vi "App - analyze RUS V6.vi"() -> ()   [LabVIEW 2021] (continued)
"mod time(min)"=58231368.86666667, "file format"=enum."binary", "power(V)"=2.1, "Magn Field(T) "=0.0}, {"temperature"=14.481, "temperature str"="14.48100", "file path"=path "D:/Data/Ultrasound/LSCO/LSCO22__130814c/5_Cooling_2nd_try/September_2014/091814/14.48100K_500_2500_2.10000V_0.00000T_Sep18-2014__06-50-12_001_091814.bin", "last mod"=timestamp(3493882212 s since 1904-01-01), "file name str"="D:\\Data\\Ultrasound\\LSCO\\LSCO22__130814c\\5_Cooling_2nd_try\\September_2014\\091814\\14.48100K_500_2500_2.10000V_0.00000T_Sep18-2014__06-50-12_001_091814.bin", "mod time(min)"=58231370.2, "file format"=enum."binary", "power(V)"=2.1, "Magn Field(T) "=0.0}, {"temperature"=14.483, "temperature str"="14.48300", "file path"=path "D:/Data/Ultrasound/LSCO/LSCO22__130814c/5_Cooling_2nd_try/September_2014/091814/14.48300K_500_2500_2.10000V_0.00000T_Sep18-2014__06-51-31_001_091814.bin", "last mod"=timestamp(3493882291 s since 1904-01-01), "file name str"="D:\\Data\\Ultrasound\\LSCO\\LSCO22__130814c\\5_Cooling_2nd_try\\September_2014\\091814\\14.48300K_500_2500_2.10000V_0.00000T_Sep18-2014__06-51-31_001_091814.bin", "mod time(min)"=58231371.516666666, "file format"=enum."binary", "power(V)"=2.1, "Magn Field(T) "=0.0}, {"temperature"=14.483, "temperature str"="14.48300", "file path"=path "D:/Data/Ultrasound/LSCO/LSCO22__130814c/5_Cooling_2nd_try/September_2014/091814/14.48300K_500_2500_2.10000V_0.00000T_Sep18-2014__06-52-50_001_091814.bin", "last mod"=timestamp(3493882370 s since 1904-01-01), "file name str"="D:\\Data\\Ultrasound\\LSCO\\LSCO22__130814c\\5_Cooling_2nd_try\\September_2014\\091814\\14.48300K_500_2500_2.10000V_0.00000T_Sep18-2014__06-52-50_001_091814.bin", "mod time(min)"=58231372.833333336, "file format"=enum."binary", "power(V)"=2.1, "Magn Field(T) "=0.0}, {"temperature"=14.484, "temperature str"="14.48400", "file path"=path "D:/Data/Ultrasound/LSCO/LSCO22__130814c/5_Cooling_2nd_try/September_2014/091814/14.48400K_500_2500_2.10000V_0.00000T_Sep18-2014__06-54-10_001_091814.bin", "last mod"=timestamp(3493882450 s since 1904-01-01), "file name str"="D:\\Data\\Ultrasound\\LSCO\\LSCO22__130814c\\5_Cooling_2nd_try\\September_2014\\091814\\14.48400K_500_2500_2.10000V_0.00000T_Sep18-2014__06-54-10_001_091814.bin", "mod time(min)"=58231374.166666664, "file format"=enum."binary", "power(V)"=2.1, "Magn Field(T) "=0.0}, {"temperature"=14.488, "temperature str"="14.48800", "file path"=path "D:/Data/Ultrasound/LSCO/LSCO22__130814c/5_Cooling_2nd_try/September_2014/091814/14.48800K_500_2500_2.10000V_0.00000T_Sep18-2014__06-55-29_001_091814.bin", "last mod"=timestamp(3493882529 s since 1904-01-01), "file name str"="D:\\Data\\Ultrasound\\LSCO\\LSCO22__130814c\\5_Cooling_2nd_try\\September_2014\\091814\\14.48800K_500_2500_2.10000V_0.00000T_Sep18-2014__06-55-29_001_091814.bin", "mod time(min)"=58231375.483333334, "file format"=enum."binary", "power(V)"=2.1, "Magn Field(T) "=0.0}, {"temperature"=14.49, "temperature str"="14.49000", "file path"=path "D:/Data/Ultrasound/LSCO/LSCO22__130814c/5_Cooling_2nd_try/September_2014/091814/14.49000K_500_2500_2.10000V_0.00000T_Sep18-2014__06-56-49_001_091814.bin", "last mod"=timestamp(3493882609 s since 1904-01-01), "file name str"="D:\\Data\\Ultrasound\\LSCO\\LSCO22__130814c\\5_Cooling_2nd_try\\September_2014\\091814\\14.49000K_500_2500_2.10000V_0.00000T_Sep18-2014__06-56-49_001_091814.bin", "mod time(min)"=58231376.81666667, "file format"=enum."binary", "power(V)"=2.1, "Magn Field(T) "=0.0}, {"temperature"=14.491, "temperature str"="14.49100", "file path"=path "D:/Data/Ultrasound/LSCO/LSCO22__130814c/5_Cooling_2nd_try/September_2014/091814/14.49100K_500_2500_2.10000V_0.00000T_Sep18-2014__06-58-08_001_091814.bin", "last mod"=timestamp(3493882688 s since 1904-01-01), "file name str"="D:\\Data\\Ultrasound\\LSCO\\LSCO22__130814c\\5_Cooling_2nd_try\\September_2014\\091814\\14.49100K_500_2500_2.10000V_0.00000T_Sep18-2014__06-58-08_001_091814.bin", "mod time(min)"=58231378.13333333, "file format"=enum."binary", "power(V)"=2.1, "Magn Field(T) "=0.0}, {"temperature"=14.493, "temperature str"="14.49300", "file path"=path "D:/Data/Ultrasound/LSCO/LSCO22__130814c/5_Cooling_2nd_try/September_2014/091814/14.49300K_500_2500_2.10000V_0.00000T_Sep18-2014__06-59-27_001_091814.bin", "last mod"=timestamp(3493882767 s since 1904-01-01), "file name str"="D:\\Data\\Ultrasound\\LSCO\\LSCO22__130814c\\5_Cooling_2nd_try\\September_2014\\091814\\14.49300K_500_2500_2.10000V_0.00000T_Sep18-2014__06-59-27_001_091814.bin", "mod time(min)"=58231379.45, "file format"=enum."binary", "power(V)"=2.1, "Magn Field(T) "=0.0}, {"temperature"=14.491, "temperature str"="14.49100", "file path"=path "D:/Data/Ultrasound/LSCO/LSCO22__130814c/5_Cooling_2nd_try/September_2014/091814/14.49100K_500_2500_2.10000V_0.00000T_Sep18-2014__07-00-47_001_091814.bin", "last mod"=timestamp(3493882847 s since 1904-01-01), "file name str"="D:\\Data\\Ultrasound\\LSCO\\LSCO22__130814c\\5_Cooling_2nd_try\\September_2014\\091814\\14.49100K_500_2500_2.10000V_0.00000T_Sep18-2014__07-00-47_001_091814.bin", "mod time(min)"=58231380.78333333, "file format"=enum."binary", "power(V)"=2.1, "Magn Field(T) "=0.0}, {"temperature"=14.489, "temperature str"="14.48900", "file path"=path "D:/Data/Ultrasound/LSCO/LSCO22__130814c/5_Cooling_2nd_try/September_2014/091814/14.48900K_500_2500_2.10000V_0.00000T_Sep18-2014__07-02-06_001_091814.bin", "last mod"=timestamp(3493882926 s since 1904-01-01), "file name str"="D:\\Data\\Ultrasound\\LSCO\\LSCO22__130814c\\5_Cooling_2nd_try\\September_2014\\091814\\14.48900K_500_2500_2.10000V_0.00000T_Sep18-2014__07-02-06_001_091814.bin", "mod time(min)"=58231382.1, "file format"=enum."binary", "power(V)"=2.1, "Magn Field(T) "=0.0}, {"temperature"=14.491, "temperature str"="14.49100", "file path"=path "D:/Data/Ultrasound/LSCO/LSCO22__130814c/5_Cooling_2nd_try/September_2014/091814/14.49100K_500_2500_2.10000V_0.00000T_Sep18-2014__07-03-26_001_091814.bin", "last mod"=timestamp(3493883006 s since 1904-01-01), "file name str"="D:\\Data\\Ultrasound\\LSCO\\LSCO22__130814c\\5_Cooling_2nd_try\\September_2014\\091814\\14.49100K_500_2500_2.10000V_0.00000T_Sep18-2014__07-03-26_001_091814.bin", "mod time(min)"=58231383.43333333, "file format"=enum."binary", "power(V)"=2.1, "Magn Field(T) "=0.0}, {"temperature"=14.492, "temperature str"="14.49200", "file path"=path "D:/Data/Ultrasound/LSCO/LSCO22__130814c/5_Cooling_2nd_try/September_2014/091814/14.49200K_500_2500_2.10000V_0.00000T_Sep18-2014__07-04-45_001_091814.bin", "last mod"=timestamp(3493883085 s since 1904-01-01), "file name str"="D:\\Data\\Ultrasound\\LSCO\\LSCO22__130814c\\5_Cooling_2nd_try\\September_2014\\091814\\14.49200K_500_2500_2.10000V_0.00000T_Sep18-2014__07-04-45_001_091814.bin", "mod time(min)"=58231384.75, "file format"=enum."binary", "power(V)"=2.1, "Magn Field(T) "=0.0}, {"temperature"=14.492, "temperature str"="14.49200", "file path"=path "D:/Data/Ultrasound/LSCO/LSCO22__130814c/5_Cooling_2nd_try/September_2014/091814/14.49200K_500_2500_2.10000V_0.00000T_Sep18-2014__07-06-04_001_091814.bin", "last mod"=timestamp(3493883164 s since 1904-01-01), "file name str"="D:\\Data\\Ultrasound\\LSCO\\LSCO22__130814c\\5_Cooling_2nd_try\\September_2014\\091814\\14.49200K_500_2500_2.10000V_0.00000T_Sep18-2014__07-06-04_001_091814.bin", "mod time(min)"=58231386.06666667, "file format"=enum."binary", "power(V)"=2.1, "Magn Field(T) "=0.0}, {"temperature"=14.496, "temperature str"="14.49600", "file path"=path "D:/Data/Ultrasound/LSCO/LSCO22__130814c/5_Cooling_2nd_try/September_2014/091814/14.49600K_500_2500_2.10000V_0.00000T_Sep18-2014__07-07-24_001_091814.bin", "last mod"=timestamp(3493883244 s since 1904-01-01), "file name str"="D:\\Data\\Ultrasound\\LSCO\\LSCO22__130814c\\5_Cooling_2nd_try\\September_2014\\091814\\14.49600K_500_2500_2.10000V_0.00000T_Sep18-2014__07-07-24_001_091814.bin", "mod time(min)"=58231387.4, "file format"=enum."binary", "power(V)"=2.1, "Magn Field(T) "=0.0}, {"temperature"=14.498, "temperature str"="14.49800", "file path"=path "D:/Data/Ultrasound/LSCO/LSCO22__130814c/5_Cooling_2nd_try/September_2014/091814/14.49800K_500_2500_2.10000V_0.00000T_Sep18-2014__07-08-43_001_091814.bin", "last mod"=timestamp(3493883323 s since 1904-01-01), "file name str"="D:\\Data\\Ultrasound\\LSCO\\LSCO22__130814c\\5_Cooling_2nd_try\\September_2014\\091814\\14.49800K_500_2500_2.10000V_0.00000T_Sep18-2014__07-08-43_001_091814.bin", "mod time(min)"=58231388.71666667, "file format"=enum."binary", "power(V)"=2.1, "Magn Field(T) "=0.0}, {"temperature"=14.495, "temperature str"="14.49500", "file path"=path "D:/Data/Ultrasound/LSCO/LSCO22__130814c/5_Cooling_2nd_try/September_2014/091814/14.49500K_500_2500_2.10000V_0.00000T_Sep18-2014__07-10-02_001_091814.bin", "last mod"=timestamp(3493883402 s since 1904-01-01), "file name str"="D:\\Data\\Ultrasound\\LSCO\\LSCO22__130814c\\5_Cooling_2nd_try\\September_2014\\091814\\14.49500K_500_2500_2.10000V_0.00000T_Sep18-2014__07-10-02_001_091814.bin", "mod time(min)"=58231390.03333333, "file format"=enum."binary", "power(V)"=2.1, "Magn Field(T) "=0.0}, {"temperature"=14.498, "temperature str"="14.49800", "file path"=path "D:/Data/Ultrasound/LSCO/LSCO22__130814c/5_Cooling_2nd_try/September_2014/091814/14.49800K_500_2500_2.10000V_0.00000T_Sep18-2014__07-11-22_001_091814.bin", "last mod"=timestamp(3493883482 s since 1904-01-01), "file name str"="D:\\Data\\Ultrasound\\LSCO\\LSCO22__130814c\\5_Cooling_2nd_try\\September_2014\\091814\\14.49800K_500_2500_2.10000V_0.00000T_Sep18-2014__07-11-22_001_091814.bin", "mod time(min)"=58231391.36666667, "file format"=enum."binary", "power(V)"=2.1, "Magn Field(T) "=0.0}, {"temperature"=14.496, "temperature str"="14.49600", "file path"=path "D:/Data/Ultrasound/LSCO/LSCO22__130814c/5_Cooling_2nd_try/September_2014/091814/14.49600K_500_2500_2.10000V_0.00000T_Sep18-2014__07-12-41_001_091814.bin", "last mod"=timestamp(3493883561 s since 1904-01-01), "file name str"="D:\\Data\\Ultrasound\\LSCO\\LSCO22__130814c\\5_Cooling_2nd_try\\September_2014\\091814\\14.49600K_500_2500_2.10000V_0.00000T_Sep18-2014__07-12-41_001_091814.bin", "mod time(min)"=58231392.68333333, "file format"=enum."binary", "power(V)"=2.1, "Magn Field(T) "=0.0}, {"temperature"=14.503, "temperature str"="14.50300", "file path"=path "D:/Data/Ultrasound/LSCO/LSCO22__130814c/5_Cooling_2nd_try/September_2014/091814/14.50300K_500_2500_2.10000V_0.00000T_Sep18-2014__07-14-01_001_091814.bin", "last mod"=timestamp(3493883641 s since 1904-01-01), "file name str"="D:\\Data\\Ultrasound\\LSCO\\LSCO22__130814c\\5_Cooling_2nd_try\\September_2014\\091814\\14.50300K_500_2500_2.10000V_0.00000T_Sep18-2014__07-14-01_001_091814.bin", "mod time(min)"=58231394.016666666, "file format"=enum."binary", "power(V)"=2.1, "Magn Field(T) "=0.0}, {"temperature"=14.504, "temperature str"="14.50400", "file path"=path "D:/Data/Ultrasound/LSCO/LSCO22__130814c/5_Cooling_2nd_try/September_2014/091814/14.50400K_500_2500_2.10000V_0.00000T_Sep18-2014__07-15-20_001_091814.bin", "last mod"=timestamp(3493883720 s since 1904-01-01), "file name str"="D:\\Data\\Ultrasound\\LSCO\\LSCO22__130814c\\5_Cooling_2nd_try\\September_2014\\091814\\14.50400K_500_2500_2.10000V_0.00000T_Sep18-2014__07-15-20_001_091814.bin", "mod time(min)"=58231395.333333336, "file format"=enum."binary", "power(V)"=2.1, "Magn Field(T) "=0.0}, {"temperature"=14.507, "temperature str"="14.50700", "file path"=path "D:/Data/Ultrasound/LSCO/LSCO22__130814c/5_Cooling_2nd_try/September_2014/091814/14.50700K_500_2500_2.10000V_0.00000T_Sep18-2014__07-16-39_001_091814.bin", "last mod"=timestamp(3493883799 s since 1904-01-01), "file name str"="D:\\Data\\Ultrasound\\LSCO\\LSCO22__130814c\\5_Cooling_2nd_try\\September_2014\\091814\\14.50700K_500_2500_2.10000V_0.00000T_Sep18-2014__07-16-39_001_091814.bin", "mod time(min)"=58231396.65, "file format"=enum."binary", "power(V)"=2.1, "Magn Field(T) "=0.0}, {"temperature"=14.507, "temperature str"="14.50700", "file path"=path "D:/Data/Ultrasound/LSCO/LSCO22__130814c/5_Cooling_2nd_try/September_2014/091814/14.50700K_500_2500_2.10000V_0.00000T_Sep18-2014__07-17-59_001_091814.bin", "last mod"=timestamp(3493883879 s since 1904-01-01), "file name str"="D:\\Data\\Ultrasound\\LSCO\\LSCO22__130814c\\5_Cooling_2nd_try\\September_2014\\091814\\14.50700K_500_2500_2.10000V_0.00000T_Sep18-2014__07-17-59_001_091814.bin", "mod time(min)"=58231397.983333334, "file format"=enum."binary", "power(V)"=2.1, "Magn Field(T) "=0.0}, {"temperature"=14.508, "temperature str"="14.50800", "file path"=path "D:/Data/Ultrasound/LSCO/LSCO22__130814c/5_Cooling_2nd_try/September_2014/091814/14.50800K_500_2500_2.10000V_0.00000T_Sep18-2014__07-19-18_001_091814.bin", "last mod"=timestamp(3493883958 s since 1904-01-01), "file name str"="D:\\Data\\Ultrasound\\LSCO\\LSCO22__130814c\\5_Cooling_2nd_try\\September_2014\\091814\\14.50800K_500_2500_2.10000V_0.00000T_Sep18-2014__07-19-18_001_091814.bin", "mod time(min)"=58231399.3, "file format"=enum."binary", "power(V)"=2.1, "Magn Field(T) "=0.0}, {"temperature"=14.507, "temperature str"="14.50700", "file path"=path "D:/Data/Ultrasound/LSCO/LSCO22__130814c/5_Cooling_2nd_try/September_2014/091814/14.50700K_500_2500_2.10000V_0.00000T_Sep18-2014__07-20-37_001_091814.bin", "last mod"=timestamp(3493884037 s since 1904-01-01), "file name str"="D:\\Data\\Ultrasound\\LSCO\\LSCO22__130814c\\5_Cooling_2nd_try\\September_2014\\091814\\14.50700K_500_2500_2.10000V_0.00000T_Sep18-2014__07-20-37_001_091814.bin", "mod time(min)"=58231400.61666667, "file format"=enum."binary", "power(V)"=2.1, "Magn Field(T) "=0.0}, {"temperature"=14.507, "temperature str"="14.50700", "file path"=path "D:/Data/Ultrasound/LSCO/LSCO22__130814c/5_Cooling_2nd_try/September_2014/091814/14.50700K_500_2500_2.10000V_0.00000T_Sep18-2014__07-21-57_001_091814.bin", "last mod"=timestamp(3493884117 s since 1904-01-01), "file name str"="D:\\Data\\Ultrasound\\LSCO\\LSCO22__130814c\\5_Cooling_2nd_try\\September_2014\\091814\\14.50700K_500_2500_2.10000V_0.00000T_Sep18-2014__07-21-57_001_091814.bin", "mod time(min)"=58231401.95, "file format"=enum."binary", "power(V)"=2.1, "Magn Field(T) "=0.0}, {"temperature"=14.508, "temperature str"="14.50800", "file path"=path "D:/Data/Ultrasound/LSCO/LSCO22__130814c/5_Cooling_2nd_try/September_2014/091814/14.50800K_500_2500_2.10000V_0.00000T_Sep18-2014__07-23-16_001_091814.bin", "last mod"=timestamp(3493884196 s since 1904-01-01), "file name str"="D:\\Data\\Ultrasound\\LSCO\\LSCO22__130814c\\5_Cooling_2nd_try\\September_2014\\091814\\14.50800K_500_2500_2.10000V_0.00000T_Sep18-2014__07-23-16_001_091814.bin", "mod time(min)"=58231403.266666666, "file format"=enum."binary", "power(V)"=2.1, "Magn Field(T) "=0.0}, {"temperature"=14.509, "temperature str"="14.50900", "file path"=path "D:/Data/Ultrasound/LSCO/LSCO22__130814c/5_Cooling_2nd_try/September_2014/091814/14.50900K_500_2500_2.10000V_0.00000T_Sep18-2014__07-24-36_001_091814.bin", "last mod"=timestamp(3493884276 s since 1904-01-01), "file name str"="D:\\Data\\Ultrasound\\LSCO\\LSCO22__130814c\\5_Cooling_2nd_try\\September_2014\\091814\\14.50900K_500_2500_2.10000V_0.00000T_Sep18-2014__07-24-36_001_091814.bin", "mod time(min)"=58231404.6, "file format"=enum."binary", "power(V)"=2.1, "Magn Field(T) "=0.0}, {"temperature"=14.511, "temperature str"="14.51100", "file path"=path "D:/Data/Ultrasound/LSCO/LSCO22__130814c/5_Cooling_2nd_try/September_2014/091814/14.51100K_500_2500_2.10000V_0.00000T_Sep18-2014__07-25-55_001_091814.bin", "last mod"=timestamp(3493884355 s since 1904-01-01), "file name str"="D:\\Data\\Ultrasound\\LSCO\\LSCO22__130814c\\5_Cooling_2nd_try\\September_2014\\091814\\14.51100K_500_2500_2.10000V_0.00000T_Sep18-2014__07-25-55_001_091814.bin", "mod time(min)"=58231405.916666664, "file format"=enum."binary", "power(V)"=2.1, "Magn Field(T) "=0.0}, {"temperature"=14.513, "temperature str"="14.51300", "file path"=path "D:/Data/Ultrasound/LSCO/LSCO22__130814c/5_Cooling_2nd_try/September_2014/091814/14.51300K_500_2500_2.10000V_0.00000T_Sep18-2014__07-27-14_001_091814.bin", "last mod"=timestamp(3493884434 s since 1904-01-01), "file name str"="D:\\Data\\Ultrasound\\LSCO\\LSCO22__130814c\\5_Cooling_2nd_try\\September_2014\\091814\\14.51300K_500_2500_2.10000V_0.00000T_Sep18-2014__07-27-14_001_091814.bin", "mod time(min)"=58231407.233333334, "file format"=enum."binary", "power(V)"=2.1, "Magn Field(T) "=0.0}, {"temperature"=14.511, "temperature str"="14.51100", "file path"=path "D:/Data/Ultrasound/LSCO/LSCO22__130814c/5_Cooling_2nd_try/September_2014/091814/14.51100K_500_2500_2.10000V_0.00000T_Sep18-2014__07-28-34_001_091814.bin", "last mod"=timestamp(3493884514 s since 1904-01-01), "file name str"="D:\\Data\\Ultrasound\\LSCO\\LSCO22__130814c\\5_Cooling_2nd_try\\September_2014\\091814\\14.51100K_500_2500_2.10000V_0.00000T_Sep18-2014__07-28-34_001_091814.bin", "mod time(min)"=58231408.56666667, "file format"=enum."binary", "power(V)"=2.1, "Magn Field(T) "=0.0}, {"temperature"=14.512, "temperature str"="14.51200", "file path"=path "D:/Data/Ultrasound/LSCO/LSCO22__130814c/5_Cooling_2nd_try/September_2014/091814/14.51200K_500_2500_2.10000V_0.00000T_Sep18-2014__07-29-53_001_091814.bin", "last mod"=timestamp(3493884593 s since 1904-01-01), "file name str"="D:\\Data\\Ultrasound\\LSCO\\LSCO22__130814c\\5_Cooling_2nd_try\\September_2014\\091814\\14.51200K_500_2500_2.10000V_0.00000T_Sep18-2014__07-29-53_001_091814.bin", "mod time(min)"=58231409.88333333, "file format"=enum."binary", "power(V)"=2.1, "Magn Field(T) "=0.0}, {"temperature"=14.512, "temperature str"="14.51200", "file path"=path "D:/Data/Ultrasound/LSCO/LSCO22__130814c/5_Cooling_2nd_try/September_2014/091814/14.51200K_500_2500_2.10000V_0.00000T_Sep18-2014__07-31-13_001_091814.bin", "last mod"=timestamp(3493884673 s since 1904-01-01), "file name str"="D:\\Data\\Ultrasound\\LSCO\\LSCO22__130814c\\5_Cooling_2nd_try\\September_2014\\091814\\14.51200K_500_2500_2.10000V_0.00000T_Sep18-2014__07-31-13_001_091814.bin", "mod time(min)"=58231411.21666667, "file format"=enum."binary", "power(V)"=2.1, "Magn Field(T) "=0.0}, {"temperature"=14.51, "temperature str"="14.51000", "file path"=path "D:/Data/Ultrasound/LSCO/LSCO22__130814c/5_Cooling_2nd_try/September_2014/091814/14.51000K_500_2500_2.10000V_0.00000T_Sep18-2014__07-32-32_001_091814.bin", "last mod"=timestamp(3493884752 s since 1904-01-01), "file name str"="D:\\Data\\Ultrasound\\LSCO\\LSCO22__130814c\\5_Cooling_2nd_try\\September_2014\\091814\\14.51000K_500_2500_2.10000V_0.00000T_Sep18-2014__07-32-32_001_091814.bin", "mod time(min)"=58231412.53333333, "file format"=enum."binary", "power(V)"=2.1, "Magn Field(T) "=0.0}, {"temperature"=14.511, "temperature str"="14.51100", "file path"=path "D:/Data/Ultrasound/LSCO/LSCO22__130814c/5_Cooling_2nd_try/September_2014/091814/14.51100K_500_2500_2.10000V_0.00000T_Sep18-2014__07-33-51_001_091814.bin", "last mod"=timestamp(3493884831 s since 1904-01-01), "file name str"="D:\\Data\\Ultrasound\\LSCO\\LSCO22__130814c\\5_Cooling_2nd_try\\September_2014\\091814\\14.51100K_500_2500_2.10000V_0.00000T_Sep18-2014__07-33-51_001_091814.bin", "mod time(min)"=58231413.85, "file format"=enum."binary", "power(V)"=2.1, "Magn Field(T) "=0.0}, {"temperature"=14.511, "temperature str"="14.51100", "file path"=path "D:/Data/Ultrasound/LSCO/LSCO22__130814c/5_Cooling_2nd_try/September_2014/091814/14.51100K_500_2500_2.10000V_0.00000T_Sep18-2014__07-35-11_001_091814.bin", "last mod"=timestamp(3493884911 s since 1904-01-01), "file name str"="D:\\Data\\Ultrasound\\LSCO\\LSCO22__130814c\\5_Cooling_2nd_try\\September_2014\\091814\\14.51100K_500_2500_2.10000V_0.00000T_Sep18-2014__07-35-11_001_091814.bin", "mod time(min)"=58231415.18333333, "file format"=enum."binary", "power(V)"=2.1, "Magn Field(T) "=0.0}, {"temperature"=14.511, "temperature str"="14.51100", "file path"=path "D:/Data/Ultrasound/LSCO/LSCO22__130814c/5_Cooling_2nd_try/September_2014/091814/14.51100K_500_2500_2.10000V_0.00000T_Sep18-2014__07-36-30_001_091814.bin", "last mod"=timestamp(3493884990 s since 1904-01-01), "file name str"="D:\\Data\\Ultrasound\\LSCO\\LSCO22__130814c\\5_Cooling_2nd_try\\September_2014\\091814\\14.51100K_500_2500_2.10000V_0.00000T_Sep18-2014__07-36-30_001_091814.bin", "mod time(min)"=58231416.5, "file format"=enum."binary", "power(V)"=2.1, "Magn Field(T) "=0.0}, {"temperature"=14.512, "temperature str"="14.51200", "file path"=path "D:/Data/Ultrasound/LSCO/LSCO22__130814c/5_Cooling_2nd_try/September_2014/091814/14.51200K_500_2500_2.10000V_0.00000T_Sep18-2014__07-37-49_001_091814.bin", "last mod"=timestamp(3493885069 s since 1904-01-01), "file name str"="D:\\Data\\Ultrasound\\LSCO\\LSCO22__130814c\\5_Cooling_2nd_try\\September_2014\\091814\\14.51200K_500_2500_2.10000V_0.00000T_Sep18-2014__07-37-49_001_091814.bin", "mod time(min)"=58231417.81666667, "file format"=enum."binary", "power(V)"=2.1, "Magn Field(T) "=0.0}, {"temperature"=14.517, "temperature str"="14.51700", "file path"=path "D:/Data/Ultrasound/LSCO/LSCO22__130814c/5_Cooling_2nd_try/September_2014/091814/14.51700K_500_2500_2.10000V_0.00000T_Sep18-2014__07-39-09_001_091814.bin", "last mod"=timestamp(3493885149 s since 1904-01-01), "file name str"="D:\\Data\\Ultrasound\\LSCO\\LSCO22__130814c\\5_Cooling_2nd_try\\September_2014\\091814\\14.51700K_500_2500_2.10000V_0.00000T_Sep18-2014__07-39-09_001_091814.bin", "mod time(min)"=58231419.15, "file format"=enum."binary", "power(V)"=2.1, "Magn Field(T) "=0.0}, {"temperature"=14.515, "temperature str"="14.51500", "file path"=path "D:/Data/Ultrasound/LSCO/LSCO22__130814c/5_Cooling_2nd_try/September_2014/091814/14.51500K_500_2500_2.10000V_0.00000T_Sep18-2014__07-40-28_001_091814.bin", "last mod"=timestamp(3493885228 s since 1904-01-01), "file name str"="D:\\Data\\Ultrasound\\LSCO\\LSCO22__130814c\\5_Cooling_2nd_try\\September_2014\\091814\\14.51500K_500_2500_2.10000V_0.00000T_Sep18-2014__07-40-28_001_091814.bin", "mod time(min)"=58231420.46666667, "file format"=enum."binary", "power(V)"=2.1, "Magn Field(T) "=0.0}, {"temperature"=14.518, "temperature str"="14.51800", "file path"=path "D:/Data/Ultrasound/LSCO/LSCO22__130814c/5_Cooling_2nd_try/September_2014/091814/14.51800K_500_2500_2.10000V_0.00000T_Sep18-2014__07-41-48_001_091814.bin", "last mod"=timestamp(3493885308 s since 1904-01-01), "file name str"="D:\\Data\\Ultrasound\\LSCO\\LSCO22__130814c\\5_Cooling_2nd_try\\September_2014\\091814\\14.51800K_500_2500_2.10000V_0.00000T_Sep18-2014__07-41-48_001_091814.bin", "mod time(min)"=58231421.8, "file format"=enum."binary", "power(V)"=2.1, "Magn Field(T) "=0.0}, {"temperature"=14.517, "temperature str"="14.51700", "file path"=path "D:/Data/Ultrasound/LSCO/LSCO22__130814c/5_Cooling_2nd_try/September_2014/091814/14.51700K_500_2500_2.10000V_0.00000T_Sep18-2014__07-43-07_001_091814.bin", "last mod"=timestamp(3493885387 s since 1904-01-01), "file name str"="D:\\Data\\Ultrasound\\LSCO\\LSCO22__130814c\\5_Cooling_2nd_try\\September_2014\\091814\\14.51700K_500_2500_2.10000V_0.00000T_Sep18-2014__07-43-07_001_091814.bin", "mod time(min)"=58231423.11666667, "file format"=enum."binary", "power(V)"=2.1, "Magn Field(T) "=0.0}, {"temperature"=14.517, "temperature str"="14.51700", "file path"=path "D:/Data/Ultrasound/LSCO/LSCO22__130814c/5_Cooling_2nd_try/September_2014/091814/14.51700K_500_2500_2.10000V_0.00000T_Sep18-2014__07-44-26_001_091814.bin", "last mod"=timestamp(3493885466 s since 1904-01-01), "file name str"="D:\\Data\\Ultrasound\\LSCO\\LSCO22__130814c\\5_Cooling_2nd_try\\September_2014\\091814\\14.51700K_500_2500_2.10000V_0.00000T_Sep18-2014__07-44-26_001_091814.bin", "mod time(min)"=58231424.43333333, "file format"=enum."binary", "power(V)"=2.1, "Magn Field(T) "=0.0}, {"temperature"=14.518, "temperature str"="14.51800", "file path"=path "D:/Data/Ultrasound/LSCO/LSCO22__130814c/5_Cooling_2nd_try/September_2014/091814/14.51800K_500_2500_2.10000V_0.00000T_Sep18-2014__07-45-46_001_091814.bin", "last mod"=timestamp(3493885546 s since 1904-01-01), "file name str"="D:\\Data\\Ultrasound\\LSCO\\LSCO22__130814c\\5_Cooling_2nd_try\\September_2014\\091814\\14.51800K_500_2500_2.10000V_0.00000T_Sep18-2014__07-45-46_001_091814.bin", "mod time(min)"=58231425.766666666, "file format"=enum."binary", "power(V)"=2.1, "Magn Field(T) "=0.0}, {"temperature"=14.518, "temperature str"="14.51800", "file path"=path "D:/Data/Ultrasound/LSCO/LSCO22__130814c/5_Cooling_2nd_try/September_2014/091814/14.51800K_500_2500_2.10000V_0.00000T_Sep18-2014__07-47-05_001_091814.bin", "last mod"=timestamp(3493885625 s since 1904-01-01), "file name str"="D:\\Data\\Ultrasound\\LSCO\\LSCO22__130814c\\5_Cooling_2nd_try\\September_2014\\091814\\14.51800K_500_2500_2.10000V_0.00000T_Sep18-2014__07-47-05_001_091814.bin", "mod time(min)"=58231427.083333336, "file format"=enum."binary", "power(V)"=2.1, "Magn Field(T) "=0.0}, {"temperature"=14.52, "temperature str"="14.52000", "file path"=path "D:/Data/Ultrasound/LSCO/LSCO22__130814c/5_Cooling_2nd_try/September_2014/091814/14.52000K_500_2500_2.10000V_0.00000T_Sep18-2014__07-48-25_001_091814.bin", "last mod"=timestamp(3493885705 s since 1904-01-01), "file name str"="D:\\Data\\Ultrasound\\LSCO\\LSCO22__130814c\\5_Cooling_2nd_try\\September_2014\\091814\\14.52000K_500_2500_2.10000V_0.00000T_Sep18-2014__07-48-25_001_091814.bin", "mod time(min)"=58231428.416666664, "file format"=enum."binary", "power(V)"=2.1, "Magn Field(T) "=0.0}, {"temperature"=14.525, "temperature str"="14.52500", "file path"=path "D:/Data/Ultrasound/LSCO/LSCO22__130814c/5_Cooling_2nd_try/September_2014/091814/14.52500K_500_2500_2.10000V_0.00000T_Sep18-2014__07-49-44_001_091814.bin", "last mod"=timestamp(3493885784 s since 1904-01-01), "file name str"="D:\\Data\\Ultrasound\\LSCO\\LSCO22__130814c\\5_Cooling_2nd_try\\September_2014\\091814\\14.52500K_500_2500_2.10000V_0.00000T_Sep18-2014__07-49-44_001_091814.bin", "mod time(min)"=58231429.733333334, "file format"=enum."binary", "power(V)"=2.1, "Magn Field(T) "=0.0}, {"temperature"=14.521, "temperature str"="14.52100", "file path"=path "D:/Data/Ultrasound/LSCO/LSCO22__130814c/5_Cooling_2nd_try/September_2014/091814/14.52100K_500_2500_2.10000V_0.00000T_Sep18-2014__07-51-03_001_091814.bin", "last mod"=timestamp(3493885863 s since 1904-01-01), "file name str"="D:\\Data\\Ultrasound\\LSCO\\LSCO22__130814c\\5_Cooling_2nd_try\\September_2014\\091814\\14.52100K_500_2500_2.10000V_0.00000T_Sep18-2014__07-51-03_001_091814.bin", "mod time(min)"=58231431.05, "file format"=enum."binary", "power(V)"=2.1, "Magn Field(T) "=0.0}, {"temperature"=14.524, "temperature str"="14.52400", "file path"=path "D:/Data/Ultrasound/LSCO/LSCO22__130814c/5_Cooling_2nd_try/September_2014/091814/14.52400K_500_2500_2.10000V_0.00000T_Sep18-2014__07-52-23_001_091814.bin", "last mod"=timestamp(3493885943 s since 1904-01-01), "file name str"="D:\\Data\\Ultrasound\\LSCO\\LSCO22__130814c\\5_Cooling_2nd_try\\September_2014\\091814\\14.52400K_500_2500_2.10000V_0.00000T_Sep18-2014__07-52-23_001_091814.bin", "mod time(min)"=58231432.38333333, "file format"=enum."binary", "power(V)"=2.1, "Magn Field(T) "=0.0}, {"temperature"=14.524, "temperature str"="14.52400", "file path"=path "D:/Data/Ultrasound/LSCO/LSCO22__130814c/5_Cooling_2nd_try/September_2014/091814/14.52400K_500_2500_2.10000V_0.00000T_Sep18-2014__07-53-42_001_091814.bin", "last mod"=timestamp(3493886022 s since 1904-01-01), "file name str"="D:\\Data\\Ultrasound\\LSCO\\LSCO22__130814c\\5_Cooling_2nd_try\\September_2014\\091814\\14.52400K_500_2500_2.10000V_0.00000T_Sep18-2014__07-53-42_001_091814.bin", "mod time(min)"=58231433.7, "file format"=enum."binary", "power(V)"=2.1, "Magn Field(T) "=0.0}, {"temperature"=14.524, "temperature str"="14.52400", "file path"=path "D:/Data/Ultrasound/LSCO/LSCO22__130814c/5_Cooling_2nd_try/September_2014/091814/14.52400K_500_2500_2.10000V_0.00000T_Sep18-2014__07-55-01_001_091814.bin", "last mod"=timestamp(3493886101 s since 1904-01-01), "file name str"="D:\\Data\\Ultrasound\\LSCO\\LSCO22__130814c\\5_Cooling_2nd_try\\September_2014\\091814\\14.52400K_500_2500_2.10000V_0.00000T_Sep18-2014__07-55-01_001_091814.bin", "mod time(min)"=58231435.016666666, "file format"=enum."binary", "power(V)"=2.1, "Magn Field(T) "=0.0}, {"temperature"=14.523, "temperature str"="14.52300", "file path"=path "D:/Data/Ultrasound/LSCO/LSCO22__130814c/5_Cooling_2nd_try/September_2014/091814/14.52300K_500_2500_2.10000V_0.00000T_Sep18-2014__07-56-21_001_091814.bin", "last mod"=timestamp(3493886181 s since 1904-01-01), "file name str"="D:\\Data\\Ultrasound\\LSCO\\LSCO22__130814c\\5_Cooling_2nd_try\\September_2014\\091814\\14.52300K_500_2500_2.10000V_0.00000T_Sep18-2014__07-56-21_001_091814.bin", "mod time(min)"=58231436.35, "file format"=enum."binary", "power(V)"=2.1, "Magn Field(T) "=0.0}, {"temperature"=14.527, "temperature str"="14.52700", "file path"=path "D:/Data/Ultrasound/LSCO/LSCO22__130814c/5_Cooling_2nd_try/September_2014/091814/14.52700K_500_2500_2.10000V_0.00000T_Sep18-2014__07-57-40_001_091814.bin", "last mod"=timestamp(3493886260 s since 1904-01-01), "file name str"="D:\\Data\\Ultrasound\\LSCO\\LSCO22__130814c\\5_Cooling_2nd_try\\September_2014\\091814\\14.52700K_500_2500_2.10000V_0.00000T_Sep18-2014__07-57-40_001_091814.bin", "mod time(min)"=58231437.666666664, "file format"=enum."binary", "power(V)"=2.1, "Magn Field(T) "=0.0}, {"temperature"=14.522, "temperature str"="14.52200", "file path"=path "D:/Data/Ultrasound/LSCO/LSCO22__130814c/5_Cooling_2nd_try/September_2014/091814/14.52200K_500_2500_2.10000V_0.00000T_Sep18-2014__07-59-00_001_091814.bin", "last mod"=timestamp(3493886340 s since 1904-01-01), "file name str"="D:\\Data\\Ultrasound\\LSCO\\LSCO22__130814c\\5_Cooling_2nd_try\\September_2014\\091814\\14.52200K_500_2500_2.10000V_0.00000T_Sep18-2014__07-59-00_001_091814.bin", "mod time(min)"=58231439.0, "file format"=enum."binary", "power(V)"=2.1, "Magn Field(T) "=0.0}, {"temperature"=14.52, "temperature str"="14.52000", "file path"=path "D:/Data/Ultrasound/LSCO/LSCO22__130814c/5_Cooling_2nd_try/September_2014/091814/14.52000K_500_2500_2.10000V_0.00000T_Sep18-2014__08-00-19_001_091814.bin", "last mod"=timestamp(3493886419 s since 1904-01-01), "file name str"="D:\\Data\\Ultrasound\\LSCO\\LSCO22__130814c\\5_Cooling_2nd_try\\September_2014\\091814\\14.52000K_500_2500_2.10000V_0.00000T_Sep18-2014__08-00-19_001_091814.bin", "mod time(min)"=58231440.31666667, "file format"=enum."binary", "power(V)"=2.1, "Magn Field(T) "=0.0}, {"temperature"=14.522, "temperature str"="14.52200", "file path"=path "D:/Data/Ultrasound/LSCO/LSCO22__130814c/5_Cooling_2nd_try/September_2014/091814/14.52200K_500_2500_2.10000V_0.00000T_Sep18-2014__08-01-38_001_091814.bin", "last mod"=timestamp(3493886498 s since 1904-01-01), "file name str"="D:\\Data\\Ultrasound\\LSCO\\LSCO22__130814c\\5_Cooling_2nd_try\\September_2014\\091814\\14.52200K_500_2500_2.10000V_0.00000T_Sep18-2014__08-01-38_001_091814.bin", "mod time(min)"=58231441.63333333, "file format"=enum."binary", "power(V)"=2.1, "Magn Field(T) "=0.0}, {"temperature"=14.526, "temperature str"="14.52600", "file path"=path "D:/Data/Ultrasound/LSCO/LSCO22__130814c/5_Cooling_2nd_try/September_2014/091814/14.52600K_500_2500_2.10000V_0.00000T_Sep18-2014__08-02-58_001_091814.bin", "last mod"=timestamp(3493886578 s since 1904-01-01), "file name str"="D:\\Data\\Ultrasound\\LSCO\\LSCO22__130814c\\5_Cooling_2nd_try\\September_2014\\091814\\14.52600K_500_2500_2.10000V_0.00000T_Sep18-2014__08-02-58_001_091814.bin", "mod time(min)"=58231442.96666667, "file format"=enum."binary", "power(V)"=2.1, "Magn Field(T) "=0.0}, {"temperature"=14.529, "temperature str"="14.52900", "file path"=path "D:/Data/Ultrasound/LSCO/LSCO22__130814c/5_Cooling_2nd_try/September_2014/091814/14.52900K_500_2500_2.10000V_0.00000T_Sep18-2014__08-04-17_001_091814.bin", "last mod"=timestamp(3493886657 s since 1904-01-01), "file name str"="D:\\Data\\Ultrasound\\LSCO\\LSCO22__130814c\\5_Cooling_2nd_try\\September_2014\\091814\\14.52900K_500_2500_2.10000V_0.00000T_Sep18-2014__08-04-17_001_091814.bin", "mod time(min)"=58231444.28333333, "file format"=enum."binary", "power(V)"=2.1, "Magn Field(T) "=0.0}, {"temperature"=14.531, "temperature str"="14.53100", "file path"=path "D:/Data/Ultrasound/LSCO/LSCO22__130814c/5_Cooling_2nd_try/September_2014/091814/14.53100K_500_2500_2.10000V_0.00000T_Sep18-2014__08-05-37_001_091814.bin", "last mod"=timestamp(3493886737 s since 1904-01-01), "file name str"="D:\\Data\\Ultrasound\\LSCO\\LSCO22__130814c\\5_Cooling_2nd_try\\September_2014\\091814\\14.53100K_500_2500_2.10000V_0.00000T_Sep18-2014__08-05-37_001_091814.bin", "mod time(min)"=58231445.61666667, "file format"=enum."binary", "power(V)"=2.1, "Magn Field(T) "=0.0}, {"temperature"=14.534, "temperature str"="14.53400", "file path"=path "D:/Data/Ultrasound/LSCO/LSCO22__130814c/5_Cooling_2nd_try/September_2014/091814/14.53400K_500_2500_2.10000V_0.00000T_Sep18-2014__08-06-56_001_091814.bin", "last mod"=timestamp(3493886816 s since 1904-01-01), "file name str"="D:\\Data\\Ultrasound\\LSCO\\LSCO22__130814c\\5_Cooling_2nd_try\\September_2014\\091814\\14.53400K_500_2500_2.10000V_0.00000T_Sep18-2014__08-06-56_001_091814.bin", "mod time(min)"=58231446.93333333, "file format"=enum."binary", "power(V)"=2.1, "Magn Field(T) "=0.0}, {"temperature"=14.533, "temperature str"="14.53300", "file path"=path "D:/Data/Ultrasound/LSCO/LSCO22__130814c/5_Cooling_2nd_try/September_2014/091814/14.53300K_500_2500_2.10000V_0.00000T_Sep18-2014__08-08-15_001_091814.bin", "last mod"=timestamp(3493886895 s since 1904-01-01), "file name str"="D:\\Data\\Ultrasound\\LSCO\\LSCO22__130814c\\5_Cooling_2nd_try\\September_2014\\091814\\14.53300K_500_2500_2.10000V_0.00000T_Sep18-2014__08-08-15_001_091814.bin", "mod time(min)"=58231448.25, "file format"=enum."binary", "power(V)"=2.1, "Magn Field(T) "=0.0}, {"temperature"=14.534, "temperature str"="14.53400", "file path"=path "D:/Data/Ultrasound/LSCO/LSCO22__130814c/5_Cooling_2nd_try/September_2014/091814/14.53400K_500_2500_2.10000V_0.00000T_Sep18-2014__08-09-35_001_091814.bin", "last mod"=timestamp(3493886975 s since 1904-01-01), "file name str"="D:\\Data\\Ultrasound\\LSCO\\LSCO22__130814c\\5_Cooling_2nd_try\\September_2014\\091814\\14.53400K_500_2500_2.10000V_0.00000T_Sep18-2014__08-09-35_001_091814.bin", "mod time(min)"=58231449.583333336, "file format"=enum."binary", "power(V)"=2.1, "Magn Field(T) "=0.0}, {"temperature"=14.532, "temperature str"="14.53200", "file path"=path "D:/Data/Ultrasound/LSCO/LSCO22__130814c/5_Cooling_2nd_try/September_2014/091814/14.53200K_500_2500_2.10000V_0.00000T_Sep18-2014__08-10-54_001_091814.bin", "last mod"=timestamp(3493887054 s since 1904-01-01), "file name str"="D:\\Data\\Ultrasound\\LSCO\\LSCO22__130814c\\5_Cooling_2nd_try\\September_2014\\091814\\14.53200K_500_2500_2.10000V_0.00000T_Sep18-2014__08-10-54_001_091814.bin", "mod time(min)"=58231450.9, "file format"=enum."binary", "power(V)"=2.1, "Magn Field(T) "=0.0}, {"temperature"=14.536, "temperature str"="14.53600", "file path"=path "D:/Data/Ultrasound/LSCO/LSCO22__130814c/5_Cooling_2nd_try/September_2014/091814/14.53600K_500_2500_2.10000V_0.00000T_Sep18-2014__08-12-13_001_091814.bin", "last mod"=timestamp(3493887133 s since 1904-01-01), "file name str"="D:\\Data\\Ultrasound\\LSCO\\LSCO22__130814c\\5_Cooling_2nd_try\\September_2014\\091814\\14.53600K_500_2500_2.10000V_0.00000T_Sep18-2014__08-12-13_001_091814.bin", "mod time(min)"=58231452.21666667, "file format"=enum."binary", "power(V)"=2.1, "Magn Field(T) "=0.0}, {"temperature"=14.538, "temperature str"="14.53800", "file path"=path "D:/Data/Ultrasound/LSCO/LSCO22__130814c/5_Cooling_2nd_try/September_2014/091814/14.53800K_500_2500_2.10000V_0.00000T_Sep18-2014__08-13-33_001_091814.bin", "last mod"=timestamp(3493887213 s since 1904-01-01), "file name str"="D:\\Data\\Ultrasound\\LSCO\\LSCO22__130814c\\5_Cooling_2nd_try\\September_2014\\091814\\14.53800K_500_2500_2.10000V_0.00000T_Sep18-2014__08-13-33_001_091814.bin", "mod time(min)"=58231453.55, "file format"=enum."binary", "power(V)"=2.1, "Magn Field(T) "=0.0}, {"temperature"=14.541, "temperature str"="14.54100", "file path"=path "D:/Data/Ultrasound/LSCO/LSCO22__130814c/5_Cooling_2nd_try/September_2014/091814/14.54100K_500_2500_2.10000V_0.00000T_Sep18-2014__08-14-52_001_091814.bin", "last mod"=timestamp(3493887292 s since 1904-01-01), "file name str"="D:\\Data\\Ultrasound\\LSCO\\LSCO22__130814c\\5_Cooling_2nd_try\\September_2014\\091814\\14.54100K_500_2500_2.10000V_0.00000T_Sep18-2014__08-14-52_001_091814.bin", "mod time(min)"=58231454.86666667, "file format"=enum."binary", "power(V)"=2.1, "Magn Field(T) "=0.0}, {"temperature"=14.544, "temperature str"="14.54400", "file path"=path "D:/Data/Ultrasound/LSCO/LSCO22__130814c/5_Cooling_2nd_try/September_2014/091814/14.54400K_500_2500_2.10000V_0.00000T_Sep18-2014__08-16-12_001_091814.bin", "last mod"=timestamp(3493887372 s since 1904-01-01), "file name str"="D:\\Data\\Ultrasound\\LSCO\\LSCO22__130814c\\5_Cooling_2nd_try\\September_2014\\091814\\14.54400K_500_2500_2.10000V_0.00000T_Sep18-2014__08-16-12_001_091814.bin", "mod time(min)"=58231456.2, "file format"=enum."binary", "power(V)"=2.1, "Magn Field(T) "=0.0}, {"temperature"=14.545, "temperature str"="14.54500", "file path"=path "D:/Data/Ultrasound/LSCO/LSCO22__130814c/5_Cooling_2nd_try/September_2014/091814/14.54500K_500_2500_2.10000V_0.00000T_Sep18-2014__08-17-31_001_091814.bin", "last mod"=timestamp(3493887451 s since 1904-01-01), "file name str"="D:\\Data\\Ultrasound\\LSCO\\LSCO22__130814c\\5_Cooling_2nd_try\\September_2014\\091814\\14.54500K_500_2500_2.10000V_0.00000T_Sep18-2014__08-17-31_001_091814.bin", "mod time(min)"=58231457.516666666, "file format"=enum."binary", "power(V)"=2.1, "Magn Field(T) "=0.0}, {"temperature"=14.542, "temperature str"="14.54200", "file path"=path "D:/Data/Ultrasound/LSCO/LSCO22__130814c/5_Cooling_2nd_try/September_2014/091814/14.54200K_500_2500_2.10000V_0.00000T_Sep18-2014__08-18-50_001_091814.bin", "last mod"=timestamp(3493887530 s since 1904-01-01), "file name str"="D:\\Data\\Ultrasound\\LSCO\\LSCO22__130814c\\5_Cooling_2nd_try\\September_2014\\091814\\14.54200K_500_2500_2.10000V_0.00000T_Sep18-2014__08-18-50_001_091814.bin", "mod time(min)"=58231458.833333336, "file format"=enum."binary", "power(V)"=2.1, "Magn Field(T) "=0.0}, {"temperature"=14.546, "temperature str"="14.54600", "file path"=path "D:/Data/Ultrasound/LSCO/LSCO22__130814c/5_Cooling_2nd_try/September_2014/091814/14.54600K_500_2500_2.10000V_0.00000T_Sep18-2014__08-20-10_001_091814.bin", "last mod"=timestamp(3493887610 s since 1904-01-01), "file name str"="D:\\Data\\Ultrasound\\LSCO\\LSCO22__130814c\\5_Cooling_2nd_try\\September_2014\\091814\\14.54600K_500_2500_2.10000V_0.00000T_Sep18-2014__08-20-10_001_091814.bin", "mod time(min)"=58231460.166666664, "file format"=enum."binary", "power(V)"=2.1, "Magn Field(T) "=0.0}, {"temperature"=14.547, "temperature str"="14.54700", "file path"=path "D:/Data/Ultrasound/LSCO/LSCO22__130814c/5_Cooling_2nd_try/September_2014/091814/14.54700K_500_2500_2.10000V_0.00000T_Sep18-2014__08-21-29_001_091814.bin", "last mod"=timestamp(3493887689 s since 1904-01-01), "file name str"="D:\\Data\\Ultrasound\\LSCO\\LSCO22__130814c\\5_Cooling_2nd_try\\September_2014\\091814\\14.54700K_500_2500_2.10000V_0.00000T_Sep18-2014__08-21-29_001_091814.bin", "mod time(min)"=58231461.483333334, "file format"=enum."binary", "power(V)"=2.1, "Magn Field(T) "=0.0}, {"temperature"=14.544, "temperature str"="14.54400", "file path"=path "D:/Data/Ultrasound/LSCO/LSCO22__130814c/5_Cooling_2nd_try/September_2014/091814/14.54400K_500_2500_2.10000V_0.00000T_Sep18-2014__08-22-48_001_091814.bin", "last mod"=timestamp(3493887768 s since 1904-01-01), "file name str"="D:\\Data\\Ultrasound\\LSCO\\LSCO22__130814c\\5_Cooling_2nd_try\\September_2014\\091814\\14.54400K_500_2500_2.10000V_0.00000T_Sep18-2014__08-22-48_001_091814.bin", "mod time(min)"=58231462.8, "file format"=enum."binary", "power(V)"=2.1, "Magn Field(T) "=0.0}, {"temperature"=14.549, "temperature str"="14.54900", "file path"=path "D:/Data/Ultrasound/LSCO/LSCO22__130814c/5_Cooling_2nd_try/September_2014/091814/14.54900K_500_2500_2.10000V_0.00000T_Sep18-2014__08-24-08_001_091814.bin", 
